vi "SavingMode.vi"() -> ()   [LabVIEW 2011]
panel:
  in  "SavingMode":T1(ring)
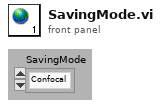
[diagram p1: front panel]
types:
  T1 = enum32{"Confocal", "HighRes", "Video", "Picture", "IntensityTrace", "Test"}
diagram:
